vi "TableControl.vi"(6 "2D Double Array":i32[][](array[numeric]), 9 "Table Control in":refnum<vi>, 10 "Arr Refnum":refnum<vi>, 11 "Table in":refnum<vi>) -> (2 "Array":string[][](array[string]))   [LabVIEW 2023]
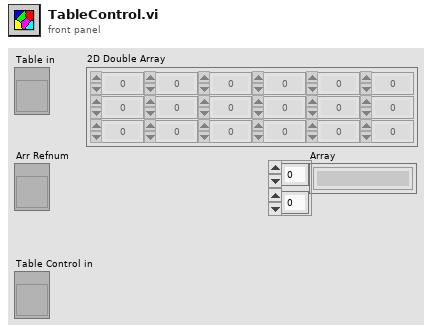
[diagram p1: front panel]
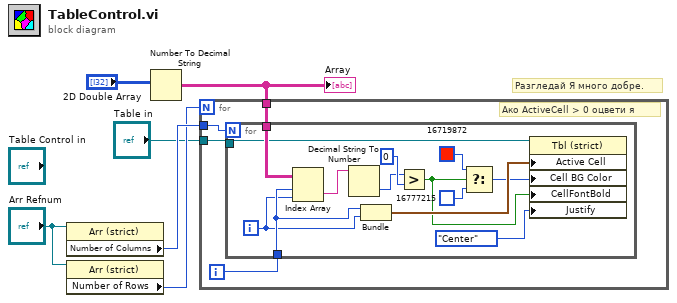
[diagram p0: block diagram]
diagram:
  # "Разгледай Я много добре."
  n1 = property on="Property Node" class="Arr (strict)"(reference="Arr Refnum") -> ("Number of Columns"=w6:u32)  [unwired: 1 in, 2 out]
  n2 = property on="Property Node" class="Arr (strict)"(reference="Arr Refnum") -> ("Number of Rows"=w5:u32)  [unwired: 1 in, 2 out]
  n3 = Number To Decimal String(number="2D Double Array") -> (decimal integer string=w4:string[][])  [unwired: 1 in]
  "Array" <- w4
  n4 = for {
    N: w5 -> [_]
    tunnel: w4 -> [w10]
    tunnel: w6 -> [w8]
    tunnel: "Table in" -> [w7]
    i -> [w9]
    # "Ако ActiveCell > 0 оцвети я"
    n5 = for {
      N: w8 -> [_]
      tunnel: w10 -> [w23]
      tunnel: w9 -> [w22]
      tunnel: w7 -> [w11]
      i -> [w21]
      n6 = Index Array "Index Array"(array=w23, index (row)=w22, index (col)=w21) -> (element=w20:string)
      n7 = Decimal String To Number(string=w20) -> (number=w12:i32)  [unwired: 2 in, 1 out]
      n8 = Bundle(w22, w21) -> (w19:cluster{i32, i32})  [unwired: 1 in]
      n9 = Greater?(x=w12, y=0) -> (0:w13:bool)
      n10 = Select(t=u32 16719872 ("Active Cell:Cell Background Color"), s=w13, f=u32 16777215 ("Active Cell:Cell Background Color")) -> (s? t:f=w16:u32)
      n11 = property on="Property Node" class="Tbl (strict)"(reference=w11, "Active Cell"=w19, "Cell BG Color"=w16, "CellFontBold"=w13, "Justify"=enum16{"Left", "Center", "Right"}."Center" ("Active Cell:Cell Justification")) -> ()  [unwired: 1 in, 2 out]
    }
  }
